vi "Main.vi"() -> ()   [LabVIEW 2015]
doc: "This template is for the Queued Message Handler design pattern.\n\nThe Event Handling Loop generates messages based on user interface actions.\n\nThe Message Handling Loop processes messages generated by the Event Handling Loop, or by other messages. The messages are string values, so new messages can be added easily to the Message Cases case structure in the Message Handling Loop. Each message cluster can also provide an optional value for Message Data, which is a variant that can be converted to whatever message-specific data is required."
uses:
  controls/UI Data.ctl
  support/Message Queue/Message Queue.lvlib
  support/User Event - Stop/User Event - Stop.lvlib
panel:
  out "Display <Replace Me>":string
  in  "Do Something Else <Replace Me>":bool
  in  "Do Something <Replace Me>":bool
  in  "Stop Button":bool
  # "These controls have associated \"Value Changed\" events configured in the Event Structure on the diagram.\n\nReplace them (and reconfigure the Event Structure) with the controls you need for your application."
  # "This template is for the Queued Message Handler design pattern.\n\nSee the block diagram for more information on how to use this template."
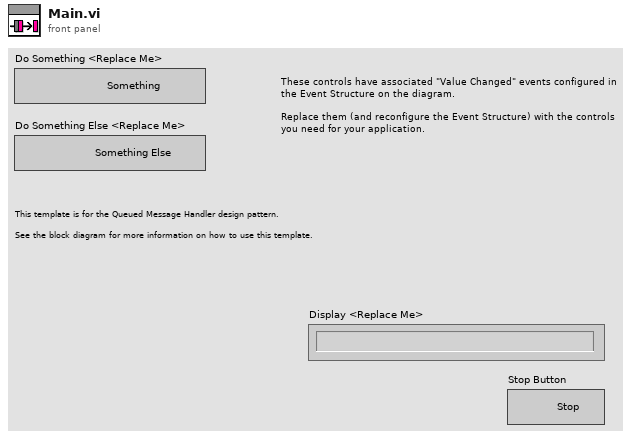
[diagram p1: front panel]
types:
  T1 = typedef "UI Data.ctl" = cluster{"Boolean <Replace Me>":bool, "String <Replace Me>":string, "Numeric <Replace Me>":dbl, "Do Something Ref":refnum<vi>, "Do Something Else Ref":refnum<vi>, "Data Display Ref":refnum<vi>, "Stop Button Ref":refnum<vi>}
  T2 = typedef "Message Queue.lvlib/All Message Queues.ctl" = cluster{"MHL":refnum<queue>, " Boiler Controller":refnum<queue>}
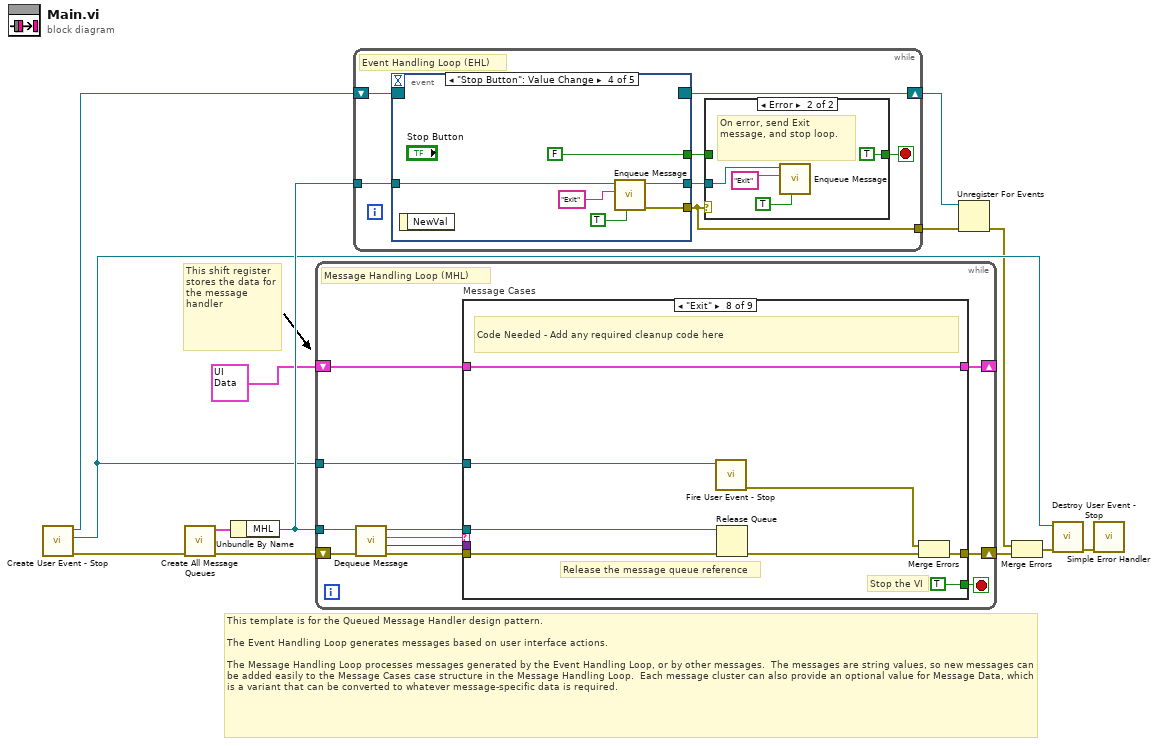
[diagram p0: block diagram]
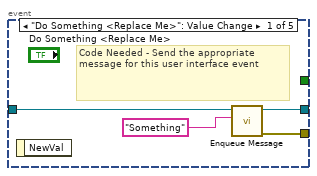
[diagram p3: hidden frame]
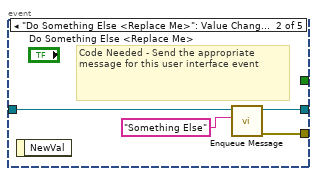
[diagram p4: hidden frame]
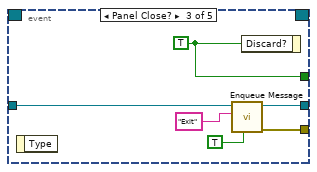
[diagram p5: hidden frame]
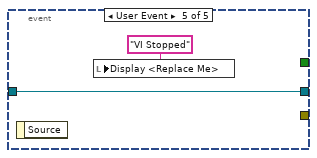
[diagram p6: hidden frame]
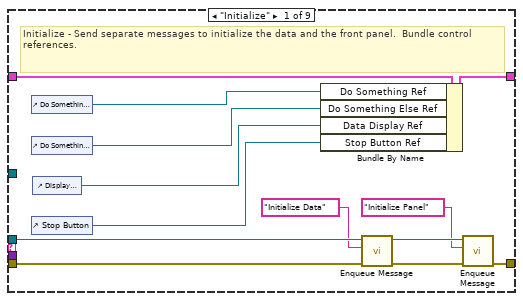
[diagram p7: hidden frame]
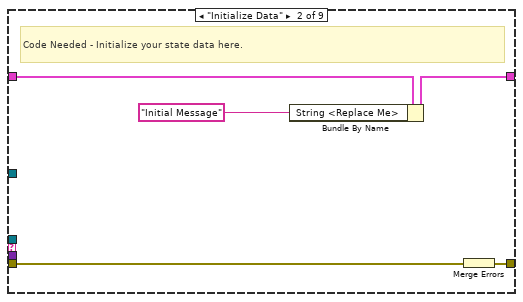
[diagram p8: hidden frame]
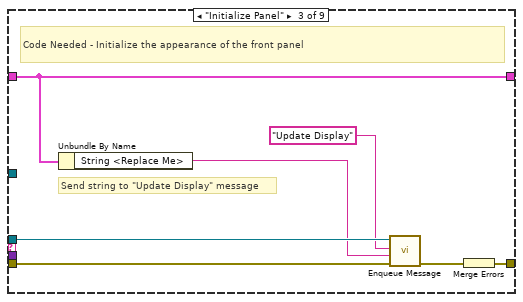
[diagram p9: hidden frame]
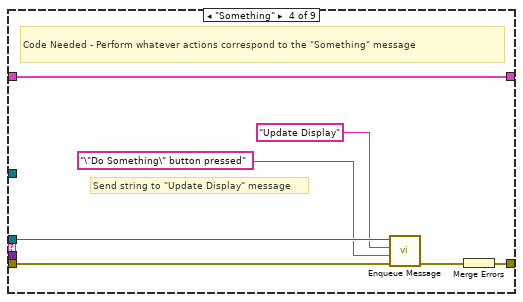
[diagram p10: hidden frame]
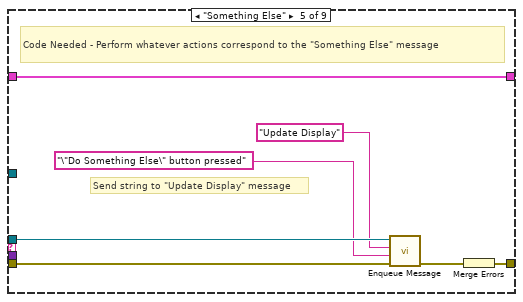
[diagram p11: hidden frame]
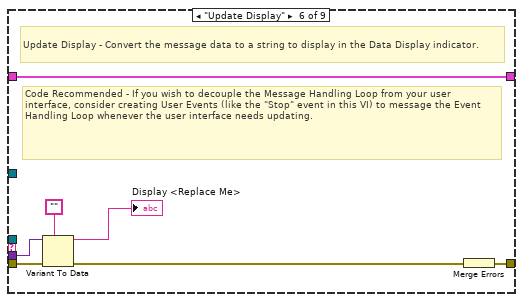
[diagram p12: hidden frame]
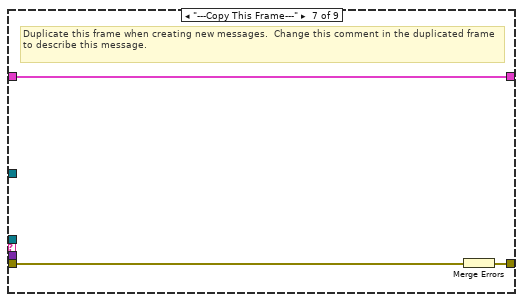
[diagram p13: hidden frame]
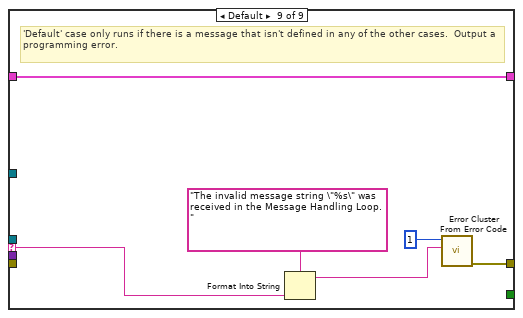
[diagram p14: hidden frame]
diagram:
  # "This template is for the Queued Message Handler design pattern.\n\nThe Event Handling Loop generates messages based on user interface actions.\n\nThe Message Handling Loop processes messages generated by the Event Handling Loop, or by other messages.  The messages are string values, so new messages can be added easily to the Message Cases case structure in the Message Handling Loop.  Each message cluster can also provide an optional value for Message Data, which is a variant that can be converted to whatever message-specific data is required."
  # "This shift register\nstores the data for the message handler"
  n1 = call "Create User Event - Stop.vi"() -> ("error out"=w9:errorcluster, "User bool - Stop"=w6:refnum<user-event>, "Event Registration Refnum"=w1:refnum<event-registration>)  [unwired: 9 in]
  n2 = call "Create All Message Queues.vi"("error in (no error)"=w9) -> ("error out"=w13:errorcluster, "Message Queues out"=w12:T2)  [unwired: 9 in]
  n3 = Unbundle By Name(w12) -> ("MHL"=w10:refnum<queue>)
  n4 = while {
    tunnel: w10 -> [w14]
    shift-right: [w23] -> _
    shift-left: T1 {"Boolean <Replace Me>"=TRUE, "String <Replace Me>"="", "Numeric <Replace Me>"=0.0, "Do Something Ref"=refnum, "Do Something Else Ref"=refnum, "Data Display Ref"=refnum, "Stop Button Ref"=refnum} ("Data Cluster") -> [w24]
    tunnel: w6 -> [w20]
    shift-right: [w21] -> w11
    shift-left: w13 -> [w19]
    stop <- w22 stop-if-true
    # "Message Handling Loop (MHL)"
    n5 = call "Dequeue Message.vi"("error in (no error)"=w19, "Message Queue"=w14) -> ("error out"=w18:errorcluster, "Message Data"=w16:variant, "Message"=w17:string, "dup Message Queue"=w15:refnum<queue>)  [unwired: 6 in]
    n6 = case "Message Cases" shown="\"Exit\"" w17 {
      selector: w17 -> [_ _ _ _ _ _ _ _ w85]
      tunnel: w15 -> [w33 _ w46 w52 w59 _ _ w81 _]
      tunnel: w18 -> [w36 w42 w47 w54 w61 w68 w73 w76 _]
      tunnel: [w37 w38 w48 w55 w62 w69 w71 w77 w83] -> w21
      tunnel: w24 -> [w30 w41 w49 w56 w63 w70 w72 w80 w87]
      tunnel: [w29 w40 w49 w56 w63 w70 w72 w80 w87] -> w23
      tunnel: [_ _ _ _ _ _ _ TRUE _] -> w22
      tunnel: w16 -> [_ _ _ _ _ w67 _ _ _]
      tunnel: w20 -> [_ _ _ _ _ _ _ w75 _]
      frame "Initialize" {
        # "Initialize - Send separate messages to initialize the data and the front panel.  Bundle control references."
        n7 = control-ref of="Do Something <Replace Me>"() -> (w28:refnum<vi>)
        n8 = control-ref of="Do Something Else <Replace Me>"() -> (w27:refnum<vi>)
        n9 = control-ref of="Stop Button"() -> (w25:refnum<vi>)
        n10 = control-ref of="Display <Replace Me>"() -> (w26:refnum<vi>)
        n11 = Bundle By Name(cluster=w30, "Do Something Ref"=w28, "Do Something Else Ref"=w27, "Data Display Ref"=w26, "Stop Button Ref"=w25) -> (w29:T1)
        n12 = call "Enqueue Message.vi"("error in (no error)"=w36, "Message"="Initialize Data", "Message Queue"=w33) -> ("error out"=w35:errorcluster, "dup Message Queue"=w34:refnum<queue>)  [unwired: 7 in]
        n13 = call "Enqueue Message.vi"("error in (no error)"=w35, "Message"="Initialize Panel", "Message Queue"=w34) -> ("error out"=w37:errorcluster)  [unwired: 7 in, 1 out]
      }
      frame "Initialize Data" {
        # "Code Needed - Initialize your state data here."
        n14 = Bundle By Name(cluster=w41, "String <Replace Me>"="Initial Message" ("Initial Message")) -> (w40:T1)
        n15 = Merge Errors(w42) -> (w38:errorcluster)
      }
      frame "Initialize Panel" {
        # "Send string to \"Update Display\" message"
        # "Code Needed - Initialize the appearance of the front panel"
        n16 = Unbundle By Name(w49) -> ("String <Replace Me>"=w43:string)
        n17 = call "Enqueue Message.vi"("error in (no error)"=w47, "Message Data"=w43, "Message"="Update Display", "Message Queue"=w46) -> ("error out"=w45:errorcluster)  [unwired: 6 in, 1 out]
        n18 = Merge Errors(w45) -> (w48:errorcluster)
      }
      frame "Something" {
        # "Send string to \"Update Display\" message"
        # "Code Needed - Perform whatever actions correspond to the \"Something\" message"
        n19 = call "Enqueue Message.vi"("error in (no error)"=w54, "Message Data"="\"Do Something\" button pressed" ("\"Do Something\" button pressed"), "Message"="Update Display", "Message Queue"=w52) -> ("error out"=w53:errorcluster)  [unwired: 6 in, 1 out]
        n20 = Merge Errors(w53) -> (w55:errorcluster)
      }
      frame "Something Else" {
        # "Send string to \"Update Display\" message"
        # "Code Needed - Perform whatever actions correspond to the \"Something Else\" message"
        n21 = call "Enqueue Message.vi"("error in (no error)"=w61, "Message Data"="\"Do Something Else\" button pressed" ("\"Do Something Else\" button pressed"), "Message"="Update Display", "Message Queue"=w59) -> ("error out"=w60:errorcluster)  [unwired: 6 in, 1 out]
        n22 = Merge Errors(w60) -> (w62:errorcluster)
      }
      frame "Update Display" {
        # "Code Recommended - If you wish to decouple the Message Handling Loop from your user interface, consider creating User Events (like the \"Stop\" event in this VI) to message the Event Handling Loop whenever the user interface needs updating."
        # "Update Display - Convert the message data to a string to display in the Data Display indicator."
        n23 = Variant To Data(error in=w68, type="", Variant=w67) -> (data=→"Display <Replace Me>":string, error out=w65:errorcluster)
        n24 = Merge Errors(w65) -> (w69:errorcluster)
      }
      frame "---Copy This Frame---" {
        # "Duplicate this frame when creating new messages.  Change this comment in the duplicated frame to describe this message."
        n25 = Merge Errors(w73) -> (w71:errorcluster)
      }
      frame "Exit" {
        # "Stop the VI"
        # "Release the message queue reference"
        # "Code Needed - Add any required cleanup code here"
        n26 = call "Fire User Event - Stop.vi"("User Event - Stop"=w75) -> ("error out"=w74:errorcluster)  [unwired: 10 in]
        n27 = Release Queue(queue=w81, error in (no error)=w76) -> (error out=w78:errorcluster)  [unwired: 1 in, 2 out]
        n28 = Merge Errors(w74, w78) -> (w77:errorcluster)
      }
      frame Default {
        # "'Default' case only runs if there is a message that isn't defined in any of the other cases.  Output a programming error."
        n29 = Format Into String(format string="The invalid message string \"%s\" was received in the Message Handling Loop." ("Unknown Message Error Text"), w85) -> (resulting string=w82:string)  [unwired: 2 in, 1 out]
        n30 = call <vilib>:"Error Cluster From Error Code.vi"("error message (\"\")"=w82, "error code (0)"=1) -> ("error out"=w83:errorcluster)  [unwired: 7 in]
      }
    }
  }
  n31 = while {
    tunnel: w10 -> [w94]
    tunnel: [w90] -> w4
    shift-right: [w89] -> w3
    shift-left: w1 -> [w88]
    stop <- w92 stop-if-true
    # "Event Handling Loop (EHL)"
    n32 = event shown="[3] \"Stop Button\": Value Change" {
      selector: w88 -> [_ _ _ _ _]
      dyn-events: [_ _ _ _ _] -> w89
      timeout: _ -> [_ _ _ _ _]
      tunnel: [_ _ w113 FALSE ("Discard?") _] -> w93
      tunnel: w94 -> [w103 w107 w112 w119 w121]
      tunnel: [w102 w105 w111 w118 _] -> w90
      tunnel: [w101 w106 w110 w116 w121] -> w91
      event "Do Something <Replace Me>": Value Change {
        # "Code Needed - Send the appropriate message for this user interface event"
        n33 = event-data() -> ()  [unwired: 1 in, 1 out]
        n34 = call "Enqueue Message.vi"("Message"="Something", "Message Queue"=w103) -> ("error out"=w102:errorcluster, "dup Message Queue"=w101:refnum<queue>)  [unwired: 8 in]
      }
      event "Do Something Else <Replace Me>": Value Change {
        # "Code Needed - Send the appropriate message for this user interface event"
        n35 = event-data() -> ()  [unwired: 1 in, 1 out]
        n36 = call "Enqueue Message.vi"("Message"="Something Else", "Message Queue"=w107) -> ("error out"=w105:errorcluster, "dup Message Queue"=w106:refnum<queue>)  [unwired: 8 in]
      }
      event Panel Close? {
        w113 = TRUE ("Discard?")
        n37 = event-data() -> ()  [unwired: 1 in, 1 out]
        n38 = call "Enqueue Message.vi"("Priority Message? (F)"=TRUE, "Message"="Exit", "Message Queue"=w112) -> ("error out"=w111:errorcluster, "dup Message Queue"=w110:refnum<queue>)  [unwired: 7 in]
        n39 = event-data("Discard?"=w113) -> ()  [unwired: 1 in, 1 out]
      }
      event "Stop Button": Value Change {
        n40 = event-data() -> ()  [unwired: 1 in, 1 out]
        n41 = call "Enqueue Message.vi"("Priority Message? (F)"=TRUE, "Message"="Exit", "Message Queue"=w119) -> ("error out"=w118:errorcluster, "dup Message Queue"=w116:refnum<queue>)  [unwired: 7 in]
      }
      event User Event {
        n42 = event-data() -> ()  [unwired: 1 in, 1 out]
        n43 = local write "Display <Replace Me>"("VI Stopped" ("VI Stopped")) -> ()
      }
    }
    n44 = case shown="Error" w90 {
      tunnel: [w95 TRUE ("Discard?")] -> w92
      tunnel: w93 -> [w95 _]
      tunnel: w91 -> [_ w98]
      frame No Error {
      }
      frame Error {
        # "On error, send Exit message, and stop loop."
        n45 = call "Enqueue Message.vi"("Priority Message? (F)"=TRUE, "Message"="Exit", "Message Queue"=w98) -> ()  [unwired: 7 in, 2 out]
      }
    }
  }
  n46 = Unregister For Events(event registration refnum=w3, error in=w4) -> (error out=w5:errorcluster)
  n47 = Merge Errors(w5, w11) -> (w7:errorcluster)
  n48 = call "Destroy User Event - Stop.vi"("error in (no error)"=w7, "User Event - Stop"=w6) -> ("error out"=w8:errorcluster)  [unwired: 9 in]
  n49 = call <vilib>:"Simple Error Handler.vi"("error in (no error)"=w8) -> ()  [unwired: 4 in, 5 out]
